vi "decodeUInt.vi"(8 "error in (no error)":errorcluster, 10 "ByteArray":u8[](array[numeric]) format="%.0x") -> (0 "error out":errorcluster, 1 "uint":u64, 2 "variant":variant, 3 "RemainingBytes":u8[](array[numeric]), 5 "Type":string)   [LabVIEW 2016, in "MsgPack.lvlib"]
uses:
  MsgPack.lvlib
  <vilib>/Utility/error.llb/Error Cluster From Error Code.vi
  <vilib>/ErrorRing/Error Ring.xnode
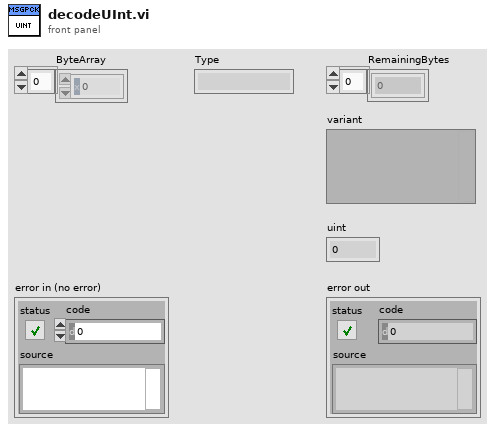
[diagram p1: front panel]
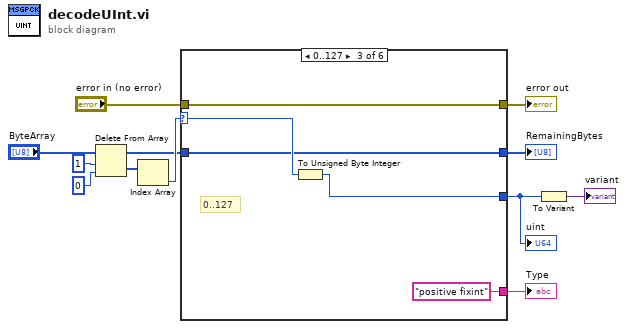
[diagram p0: block diagram]
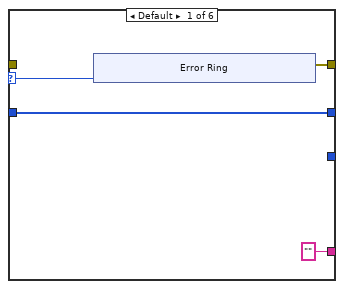
[diagram p2: hidden frame]
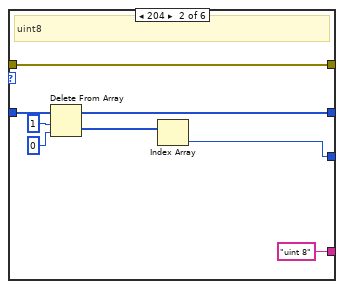
[diagram p3: hidden frame]
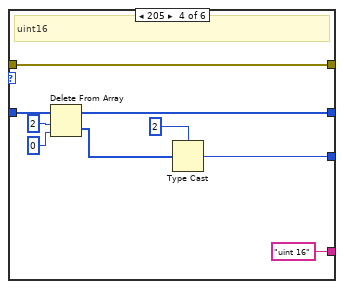
[diagram p4: hidden frame]
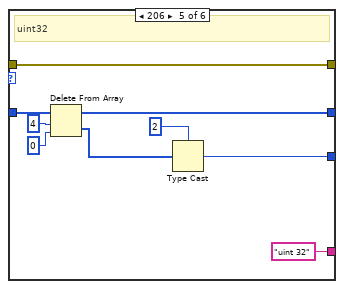
[diagram p5: hidden frame]
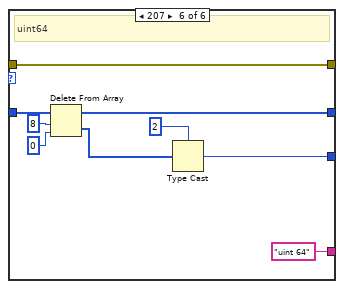
[diagram p6: hidden frame]
diagram:
  n1 = Delete From Array(array="ByteArray", length=1, index=0) -> (deleted portion=w5:u8[], array with subset deleted=w3:u8[])
  n2 = Index Array(array=w5) -> (element=w9:u8)  [unwired: 1 in]
  n3 = case shown="0..127" w9 {
    selector: w9 -> [w14 _ w36 _ _ _]
    tunnel: [w15 w31 w32 w45 w54 w63] -> w11
    tunnel: "error in (no error)" -> [_ w31 w32 w45 w54 w63]
    tunnel: ["" "uint 8" "positive fixint" "uint 16" "uint 32" "uint 64"] -> w8
    tunnel: [_ w29 w35 w43 w52 w61] -> w7
    tunnel: w3 -> [w13 w28 w34 w41 w49 w59]
    tunnel: [w13 w25 w34 w38 w47 w56] -> w2
    frame Default {
      n4 = xnode "Error Ring"("parameter 0"=w14) -> ("error out"=w15:errorcluster)
    }
    frame 204 {
      # "uint8"
      n5 = Delete From Array(array=w28, length=1, index=0) -> (deleted portion=w26:u8[], array with subset deleted=w25:u8[])
      n6 = Index Array(array=w26) -> (element=w29:u8)  [unwired: 1 in]
    }
    frame 0..127 {
      # "0..127"
      n7 = To Unsigned Byte Integer(number=w36) -> (unsigned 8bit integer=w35:u8)
    }
    frame 205 {
      # "uint16"
      n8 = Delete From Array(array=w41, length=2, index=0) -> (deleted portion=w39:u8[], array with subset deleted=w38:u8[])
      n9 = Type Cast(type=u16 2 ("length"), x=w39) -> (*(type *) &x=w43:u16)
    }
    frame 206 {
      # "uint32"
      n10 = Delete From Array(array=w49, length=4, index=0) -> (deleted portion=w48:u8[], array with subset deleted=w47:u8[])
      n11 = Type Cast(type=u32 2 ("length"), x=w48) -> (*(type *) &x=w52:u32)
    }
    frame 207 {
      # "uint64"
      n12 = Delete From Array(array=w59, length=8, index=0) -> (deleted portion=w57:u8[], array with subset deleted=w56:u8[])
      n13 = Type Cast(type=u64 2 ("length"), x=w57) -> (*(type *) &x=w61:u64)
    }
  }
  "error out" <- w11
  "Type" <- w8
  "uint" <- w7
  "RemainingBytes" <- w2
  n14 = To Variant(anything=w7) -> (Variant=→"variant":variant)
